vi "SetTrigger_mode.vi"(8 "error in (no error)":errorcluster, 10 "trigger_mode":bool, 11 "WinX32Settings in":refnum<class "WinX32Settings.lvclass">) -> (0 "error out":errorcluster, 3 "WinX32Settings out":refnum<class "WinX32Settings.lvclass">)   [LabVIEW 2011, in "Tools.lvlib" / "Settings.lvlib" / "WinX32Settings.lvclass"]
uses:
  WinX32Settings.lvclass
  CamaraSettings.lvclass
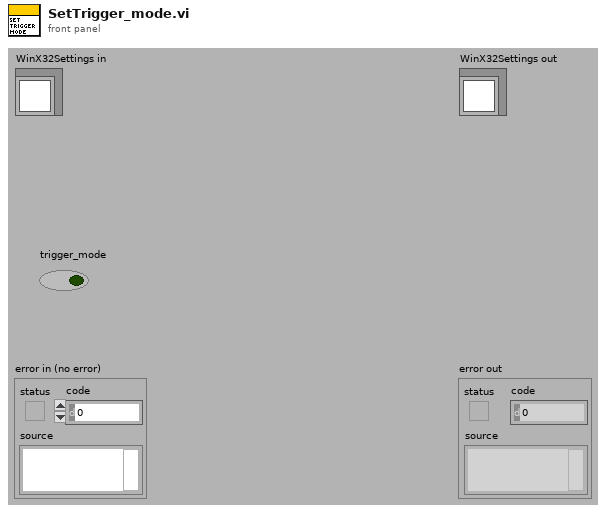
[diagram p1: front panel]
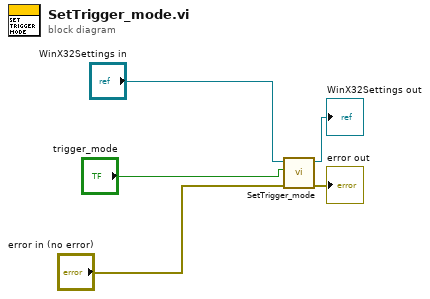
[diagram p0: block diagram]
diagram:
  n1 = call-parent "SetTrigger_mode.vi"("error in (no error)"="error in (no error)", "trigger_mode"="trigger_mode", "CamaraSettings in"="WinX32Settings in") -> ("error out"=→"error out":errorcluster, "CamaraSettings out"=→"WinX32Settings out":refnum<class "WinX32Settings.lvclass">)  [unwired: 7 in]
